vi "ep_Time to FXP.vi"(7 "operate?":bool, 8 "error in (no error)":errorcluster, 11 "time":dbl) -> (0 "error out":errorcluster, 3 "time":dbl)   [LabVIEW 2012, in "NI_EP_Protection.lvlib"]
uses:
  <vilib>/addons/Electrical Power/Protection/NI_EP_Protection.lvlib
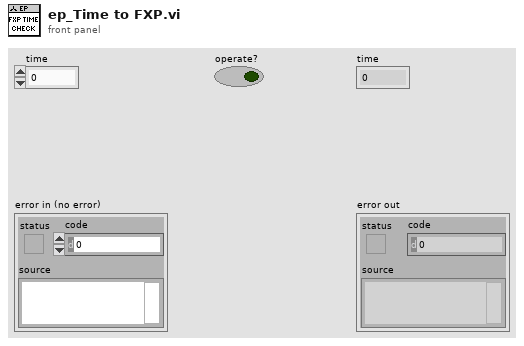
[diagram p1: front panel]
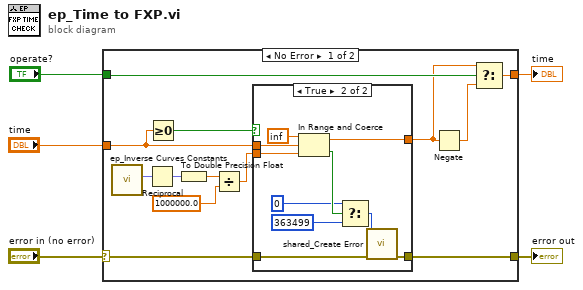
[diagram p0: block diagram]
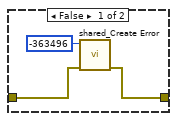
[diagram p2: hidden frame]
diagram:
  n1 = case shown="No Error" "error in (no error)" {
    selector: "error in (no error)" -> [w15 w32]
    tunnel: "time" -> [w17 _]
    tunnel: [w16 w32] -> w4
    tunnel: [w12 _] -> w3
    tunnel: "operate?" -> [w11 _]
    frame No Error {
      n2 = call <vilib>:"ep_Inverse Curves Constants.vi"() -> ("1/time"=w14:fxp<+/-,30,-10>)  [unwired: 6 in, 5 out]
      n3 = Reciprocal(x=w14) -> (1/x=w18:fxp<+/-,32,42>)
      n4 = Greater Or Equal To 0?(x=w17) -> (x >= 0?=w13:bool)
      n5 = To Double Precision Float(number=w18) -> (double precision float=w8:dbl)
      n6 = Divide(x=w8, y=1000000.0) -> (x/y=w6:dbl)
      n7 = case shown="True" w13 {
        tunnel: [_ w31] -> w9
        tunnel: w17 -> [_ w29]
        tunnel: w15 -> [w21 w28]
        tunnel: [w19 w27] -> w16
        tunnel: w6 -> [_ w22]
        frame False {
          n8 = call <vilib>:"shared_Create Error.vi"("error in (no error)"=w21, "error code (0)"=-363496) -> ("error out"=w19:errorcluster)  [unwired: 9 in]
        }
        frame True {
          n9 = In Range and Coerce(upper limit=inf, x=w29, lower limit=w22) -> (coerced(x)=w31:dbl, In Range?=w26:bool)
          n10 = Select(t=0, s=w26, f=363499 ("error code (0)")) -> (s? t:f=w25:i32)
          n11 = call <vilib>:"shared_Create Error.vi"("error in (no error)"=w28, "error code (0)"=w25) -> ("error out"=w27:errorcluster)  [unwired: 9 in]
        }
      }
      n12 = Negate(x=w9) -> (-x=w10:dbl)
      n13 = Select(t=w9, s=w11, f=w10) -> (s? t:f=w12:dbl)
    }
    frame Error {
    }
  }
  "error out" <- w4
  "time" <- w3
